vi "Database.Handler-ReconnectOne.vi"(8 "error in":errorcluster, 11 "ClientIdx":i32) -> (0 "error out":errorcluster)   [LabVIEW 2016]
uses:
  Database.Handler.Action.ctl
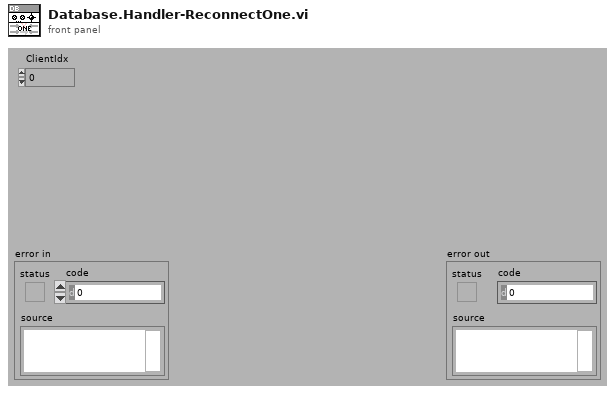
[diagram p1: front panel]
types:
  T1 = typedef "Database.Handler.Action.ctl" = enum32{"idle", "constructor", "destructor", "--- DB.Handler ---", "Setup", "Reconnect", "ReconnectAll", "ReconnectOne", "ExportData"}
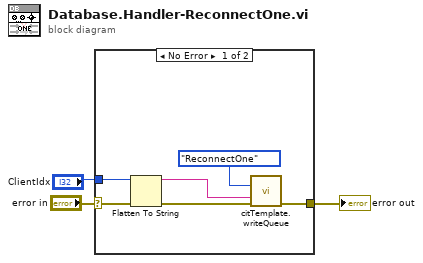
[diagram p0: block diagram]
diagram:
  n1 = case shown="No Error" "error in" {
    selector: "error in" -> [w8 w10]
    tunnel: [w9 w10] -> w2
    tunnel: "ClientIdx" -> [w4 _]
    frame No Error {
      n2 = Flatten To String(anything=w4, error in (no error)=w8) -> (data string=w5:string, error out=w6:errorcluster)  [unwired: 2 in, 1 out]
      n3 = call "citTemplate.writeQueue.vi"("event in (if not connected:all statemachine with data event)"=Database.Handler.Action."ReconnectOne" ("Action"), "data in"=w5, "error in (no error)"=w6) -> ("error out"=w9:errorcluster)  [unwired: 12 in]
    }
    frame Error {
    }
  }
  "error out" <- w2
